vi "Upload Record (S16).vi"(0 "Instrument Handle In":i32, 1 "Count":i32, 2 "Time Interval":dbl, 3 "Time Offset":dbl, 5 "Ref Channel":i32(ring) caption="Channel" items=["Calc Channel 1", "Calc Channel 2", "Calc Channel 3", "Calc Channel 4", "Ref Channel 1", "Ref Channel 2", "Ref Channel 3", "Ref Channel 4"], 7 "Type":i32, 9 "Points":u32, 11 "error in":errorcluster, 12 "Waveform":i16[](array[numeric]), 13 "Voltage Interval":dbl, 14 "Voltage Offset":dbl) -> (4 "Instrument Handle Out":i32, 15 "error out":errorcluster)   [LabVIEW 8.6, in "ZTScopeM.lvlib"]
doc: "Read the waveform in the source channel. The returned data format depends on the Transfer Type. Use \"Read Waveform Preamble\" to get the appropriate time and magnitude bases."
uses:
  ZTScopeM.lvlib
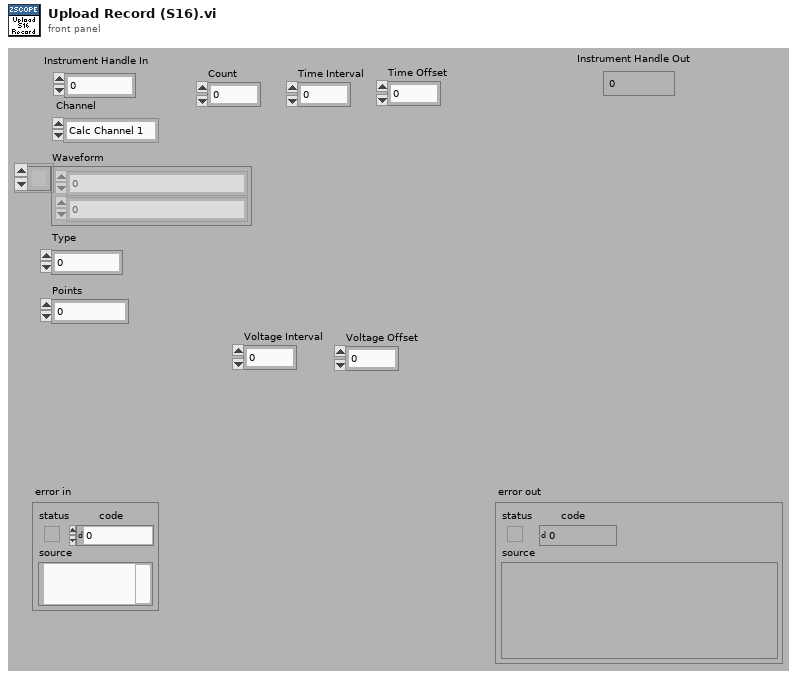
[diagram p1: front panel]
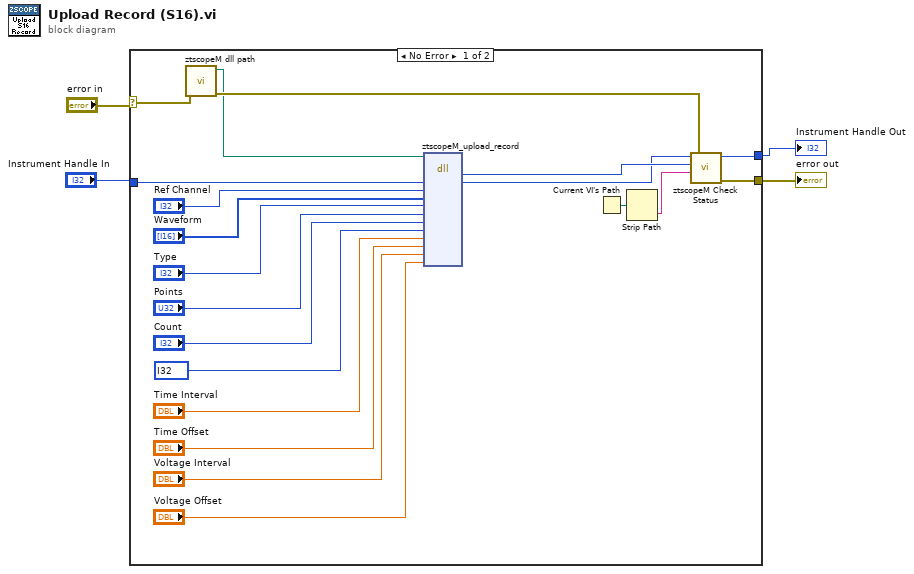
[diagram p0: block diagram]
diagram:
  n1 = case shown="No Error" "error in" {
    selector: "error in" -> [w15 w26]
    tunnel: [w19 w26] -> w1
    tunnel: "Instrument Handle In" -> [w18 w25]
    tunnel: [w20 w25] -> w3
    frame #0 {
      w10 = i32 ? items=["s8", "s16", "s32", "f32", "f64"] ("Transfer Type")
      n2 = call "ztscopeM dll path.vi"("error in (no error)"=w15) -> ("error out"=w16:errorcluster, "<instrument>.dll path"=w14:path)  [unwired: 9 in]
      n3 = dll-call lib="C:/Projects/codedepot/Teradyne/2016-1034 Teradyne ZScope API/Software/Validation/C/bin/ztscopeM Log3.dll" fn="ztscopeM_upload_record"(path in=w14, "instrumentHandle"=w18, "ref_channel"="Ref Channel", "Waveform"="Waveform", "type"="Type", "points"="Points", "count"="Count", "transferType"=w10, "time_interval"="Time Interval", "time_offset"="Time Offset", "voltage_interval"="Voltage Interval", "voltage_offset"="Voltage Offset") -> ("return type"=w22:i32, "instrumentHandle"=w21:i32)  [unwired: 12 in, 2 out]
      n4 = Current VI's Path() -> (path=w24:path)
      n5 = Strip Path(path=w24) -> (name=w23:string)  [unwired: 1 out]
      n6 = call "ztscopeM Check Status.vi"("error in"=w16, "name of VI"=w23, "status (return code)"=w22, "instrument handle in"=w21) -> ("error out"=w19:errorcluster, "instrument handle out"=w20:i32)  [unwired: 2 in]
    }
    frame #1 {
    }
  }
  "Instrument Handle Out" <- w3
  "error out" <- w1
